vi "Disconnect Mappings.vi"(8 "error in (no error)":errorcluster, 11 "Loop Data":T1) -> (0 "error out":errorcluster, 3 "Loop Data out":T1)   [LabVIEW 2016, in "System Mapping Tool.lvlib"]
uses:
  System Mapping Tool.lvlib
  TypeDefs/Loop Data.ctl
  TypeDefs/UI Refs.ctl
  NationalInstruments.VeriStand.SystemDefinitionAPI
  NationalInstruments.VeriStand.SystemStorageUI
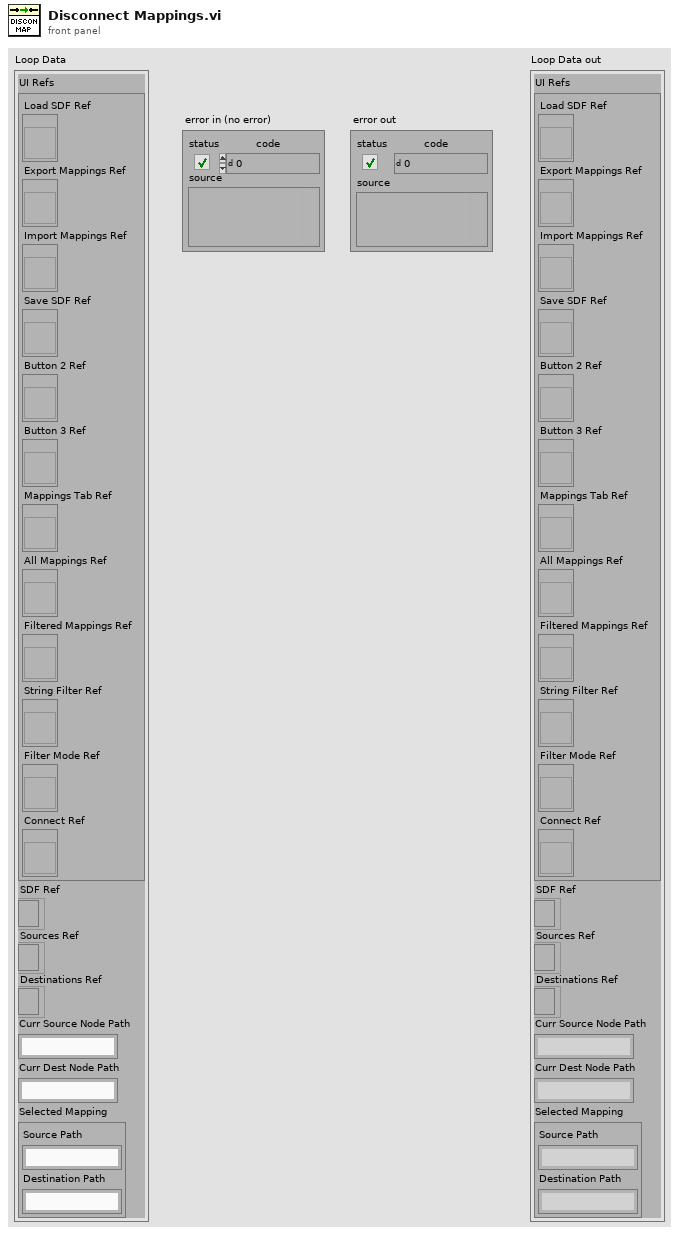
[diagram p1: front panel]
types:
  T1 = typedef "System Mapping Tool.lvlib/Loop Data.ctl" = cluster{"UI Refs":T2, "SDF Ref":refnum<k24>, "Sources Ref":refnum<k24>, "Destinations Ref":refnum<k24>, "Curr Source Node Path":string, "Curr Dest Node Path":string, "Selected Mapping":cluster{"Source Path":string, "Destination Path":string}}
  T2 = typedef "System Mapping Tool.lvlib/UI Refs.ctl" = cluster{"Load SDF Ref":refnum<vi>, "Export Mappings Ref":refnum<vi>, "Import Mappings Ref":refnum<vi>, "Save SDF Ref":refnum<vi>, "Button 2 Ref":refnum<vi>, "Button 3 Ref":refnum<vi>, "Mappings Tab Ref":refnum<vi>, "All Mappings Ref":refnum<vi>, "Filtered Mappings Ref":refnum<vi>, "String Filter Ref":refnum<vi>, "Filter Mode Ref":refnum<vi>, "Connect Ref":refnum<vi>}
  T3 = cluster{"Source Path":string, "Destination Path":string}
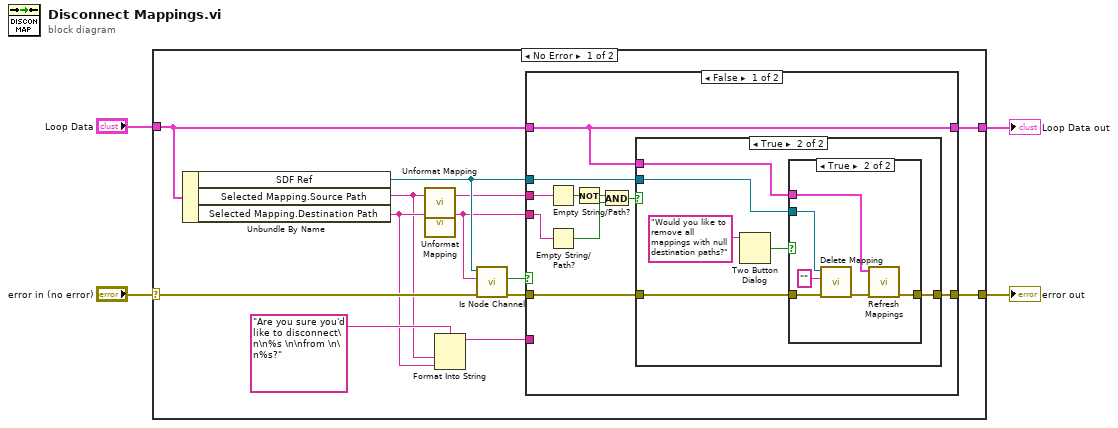
[diagram p0: block diagram]
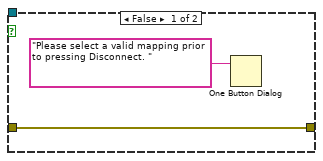
[diagram p2: hidden frame]
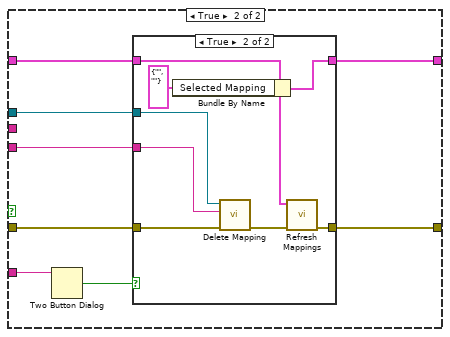
[diagram p4: hidden frame]
diagram:
  n1 = case shown="No Error" "error in (no error)" {
    selector: "error in (no error)" -> [w16 w62]
    tunnel: [w10 w62] -> w3
    tunnel: "Loop Data" -> [w14 w61]
    tunnel: [w9 w61] -> w1
    frame No Error {
      n2 = Unbundle By Name(w14) -> ("SDF Ref"=w13:refnum<k24>, "Selected Mapping.Source Path"=w6:string, "Selected Mapping.Destination Path"=w7:string)
      n3 = call "Unformat Mapping.vi"("Formatted Mapping"=w6) -> ("Mapping Path"=w8:string)  [unwired: 2 in]
      n4 = call "Unformat Mapping.vi"("Formatted Mapping"=w7) -> ("Mapping Path"=w5:string)  [unwired: 2 in]
      n5 = Format Into String(format string="Are you sure you'd like to disconnect\n\n%s \n\nfrom \n\n%s?", w6, w7) -> (resulting string=w11:string)  [unwired: 2 in, 1 out]
      n6 = call "Is Node Channel.vi"("error in (no error)"=w16, "Node Path"=w5, "SDF Ref"=w13) -> ("error out"=w15:errorcluster, "Is Channel?"=w12:bool)  [unwired: 7 in]
      n7 = case shown="False" w12 {
        tunnel: w15 -> [w22 w50]
        tunnel: w14 -> [w18 w49]
        tunnel: w13 -> [w20 w48]
        tunnel: w5 -> [w27 w47]
        tunnel: w11 -> [_ w45]
        tunnel: [w19 w44] -> w10
        tunnel: [w18 w43] -> w9
        tunnel: w8 -> [w26 _]
        frame False {
          n8 = Empty String/Path?(string/path=w26) -> (empty?=w24:bool)
          n9 = Empty String/Path?(string/path=w27) -> (empty?=w25:bool)
          n10 = Not(x=w24) -> (.not. x?=w23:bool)
          n11 = And(x=w23, y=w25) -> (x .and. y?=w21:bool)
          n12 = case shown="True" w21 {
            tunnel: w22 -> [w29 w33]
            tunnel: w20 -> [_ w32]
            tunnel: [w29 w31] -> w19
            tunnel: w18 -> [_ w30]
            frame False {
              n13 = One Button Dialog(message="Please select a valid mapping prior to pressing Disconnect. ") -> ()  [unwired: 1 in, 1 out]
            }
            frame True {
              n14 = Two Button Dialog(message="Would you like to remove all mappings with null destination paths?") -> (T button?=w34:bool)  [unwired: 2 in]
              n15 = case shown="True" w34 {
                tunnel: w33 -> [w36 w42]
                tunnel: w32 -> [_ w41]
                tunnel: [w36 w38] -> w31
                tunnel: w30 -> [_ w37]
                frame False {
                }
                frame True {
                  n16 = call "Delete Mapping.vi"("error in (no error)"=w42, "Destination Path"="", "SDF Ref"=w41) -> ("error out"=w39:errorcluster)  [unwired: 8 in]
                  n17 = call "Refresh Mappings.vi"("error in (no error)"=w39, "Loop Data"=w37) -> ("error out"=w38:errorcluster)  [unwired: 9 in]
                }
              }
            }
          }
        }
        frame True {
          n18 = Two Button Dialog(message=w45) -> (T button?=w46:bool)  [unwired: 2 in]
          n19 = case shown="True" w46 {
            tunnel: w48 -> [_ w59]
            tunnel: w50 -> [w52 w60]
            tunnel: [w52 w54] -> w44
            tunnel: w47 -> [_ w58]
            tunnel: w49 -> [w51 w53]
            tunnel: [w51 w56] -> w43
            frame False {
            }
            frame True {
              n20 = Bundle By Name(cluster=w53, "Selected Mapping"=T3 {"Source Path"="", "Destination Path"=""}) -> (w56:T1)
              n21 = call "Delete Mapping.vi"("error in (no error)"=w60, "Destination Path"=w58, "SDF Ref"=w59) -> ("error out"=w55:errorcluster)  [unwired: 8 in]
              n22 = call "Refresh Mappings.vi"("error in (no error)"=w55, "Loop Data"=w53) -> ("error out"=w54:errorcluster)  [unwired: 9 in]
            }
          }
        }
      }
    }
    frame Error {
    }
  }
  "error out" <- w3
  "Loop Data out" <- w1
